vi "boolean_run_tilt_stage.vi"(1 "loop iteration":dbl, 2 "Tot Stage Arr":dbl[](array[numeric]), 3 "number of files":dbl) -> (0 "run tilt stage":bool)   [LabVIEW 2016]
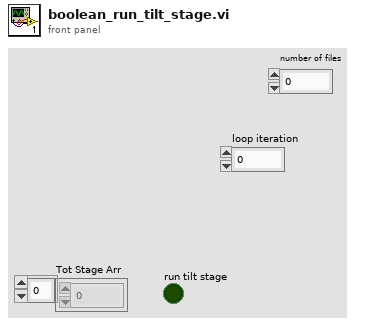
[diagram p1: front panel]
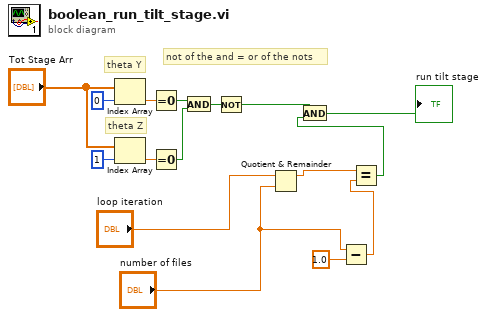
[diagram p0: block diagram]
diagram:
  # "not of the and = or of the nots"
  # "theta Z"
  # "theta Y"
  n1 = Index Array(array="Tot Stage Arr", index=0 ("index (row)")) -> (element=w13:dbl)
  n2 = Index Array(array="Tot Stage Arr", index=1 ("index (row)")) -> (element=w12:dbl)
  n3 = Equal To 0?(x=w13) -> (x = 0?=w11:bool)
  n4 = Equal To 0?(x=w12) -> (x = 0?=w10:bool)
  n5 = And(x=w11, y=w10) -> (x .and. y?=w9:bool)
  n6 = Not(x=w9) -> (.not. x?=w8:bool)
  n7 = Quotient & Remainder(x="loop iteration", y="number of files") -> (x-y*floor(x/y)=w2:dbl)  [unwired: 1 out]
  n8 = Subtract(x="number of files", y=1.0) -> (x-y=w3:dbl)
  n9 = Equal?(x=w2, y=w3) -> (x = y?=w1:bool)
  n10 = And(x=w8, y=w1) -> (x .and. y?=→"run tilt stage":bool)
